vi "CSM - Module VI Ref.vi"(6 "Response Timeout(5000ms)":i32=5000, 7 "Target Module":string="A", 8 "Error In (no error)":errorcluster) -> (0 "error out":errorcluster, 3 "CSM VI Ref":refnum<vi>)   [LabVIEW 2017, in "API String Arguments Support.lvlib"]
uses:
  API String Arguments Support.lvlib
  <userlib>/_NEVSTOP/Communicable State Machine(CSM)/_Support/Priority Queue/Priority Queue.lvclass/Priority Queue.ctl
  <userlib>/_NEVSTOP/Communicable State Machine(CSM)/_Support/Process/CSMP-Sync Call.vi
  <userlib>/_NEVSTOP/Communicable State Machine(CSM)/Utility/uuid.vi
  <userlib>/_NEVSTOP/Communicable State Machine(CSM)/Utility/Trim Both Whitespace.vi
  <userlib>/_NEVSTOP/Communicable State Machine(CSM)/_Support/CSMQ/_CSMObj-Message Check.vi
  <userlib>/_NEVSTOP/Communicable State Machine(CSM)/_Support/CSMQ/_CSMObj-Enqueue Cross-Module Message.vi
  <userlib>/_NEVSTOP/Communicable State Machine(CSM)/_Support/CSMQ/_CSMOFGV Get.vi
  <userlib>/_NEVSTOP/Communicable State Machine(CSM)/_Support/Priority Queue/Enqueue Element.vi
  <userlib>/_NEVSTOP/Communicable State Machine(CSM)/Utility/Build Error Cluster.vi
  <userlib>/_NEVSTOP/Communicable State Machine(CSM)/_Support/CSMQ/_CSMOFGV.vi
  <userlib>/_NEVSTOP/Communicable State Machine(CSM)/Communicable State Machine.lvlib
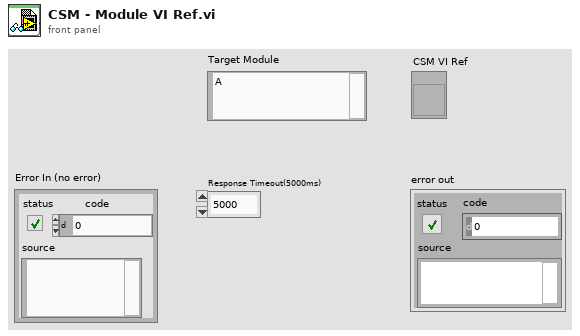
[diagram p1: front panel]
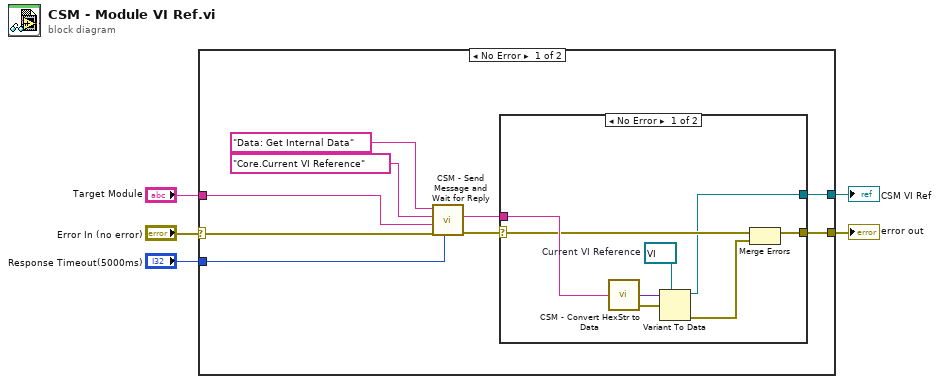
[diagram p0: block diagram]
diagram:
  n1 = case shown="No Error" "Error In (no error)" {
    selector: "Error In (no error)" -> [w9 w24]
    tunnel: "Response Timeout(5000ms)" -> [w13 _]
    tunnel: [w10 w24] -> w4
    tunnel: [w7 _] -> w2
    tunnel: "Target Module" -> [w6 _]
    frame No Error {
      n2 = call <userlib>:"CSM - Send Message and Wait for Reply.vi"("Response Timeout(5000ms)"=w13, "Error In (no error)"=w9, "Target Module"=w6, "Arguments (\"\")"="Core.Current VI Reference" ("Name(\"\" to use uuid)"), "State"="Data: Get Internal Data") -> ("error out"=w11:errorcluster, "Arguments"=w12:string)  [unwired: 4 in, 1 out]
      n3 = case shown="No Error" w11 {
        selector: w11 -> [w17 w23]
        tunnel: w12 -> [w22 _]
        tunnel: [w18 w23] -> w10
        tunnel: [w15 _] -> w7
        frame No Error {
          w19 = refnum<vi> refnum  # Current VI Reference
          n4 = call <userlib>:"CSM - Convert HexStr to Data.vi"("HEX String"=w22) -> ("Variant"=w20:variant, "error out"=w21:errorcluster)  [unwired: 7 in]
          n5 = Variant To Data(error in=w21, type=w19, Variant=w20) -> (data=w15:refnum<vi>, error out=w16:errorcluster)
          n6 = Merge Errors(w17, w16) -> (w18:errorcluster)
        }
        frame Error {
        }
      }
    }
    frame Error {
    }
  }
  "error out" <- w4
  "CSM VI Ref" <- w2
